vi "BRAM_ReadScoreNumbers.vi"(1 "Number":i16, 4 "Address":i16) -> (16 "PixelData":fxp<+,4,4>)   [LabVIEW 2018]
uses:
  <vilib>/rvi/Memory/Memory_Emulation/nirvimemoryFastEmulation.vi
  <vilib>/rvi/Memory/Memory_Emulation/nirvimemoryEmulation.vi
  <vilib>/rvi/Emulation/niFpgaEmulationIsFPGAContextNoSignature.vi
  <vilib>/rvi/DataTransferAndStorage/Container/Common/niFpgaContainerGetUniqueNameForEmu.vi
  <vilib>/rvi/Emulation/niFpgaProcessEmulError.vi
  <vilib>/rvi/Emulation/niFpgaSctlEmulationGetInTimedLoop.vi
  <vilib>/rvi/errors/nirviReportUnexpectedCaseInternalError (U32).vi
  <vilib>/rvi/DataTransferAndStorage/Container/XNode/niFpgaContainer.xnode
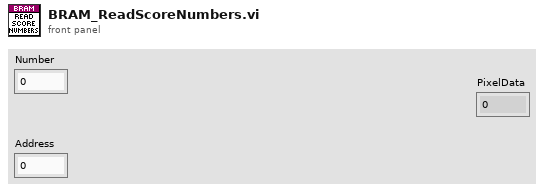
[diagram p1: front panel]
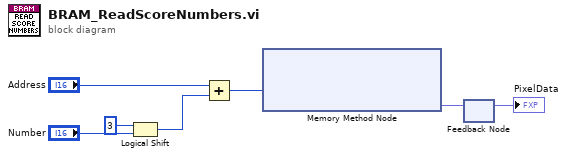
[diagram p0: block diagram]
diagram:
  n1 = Logical Shift(y=i16 3, x="Number") -> (x << y=w1:i16)
  n2 = Add(x="Address", y=w1) -> (x+y=w4:i16)
  n3 = xnode ("Memory Method Node")("Address A"=w4) -> ("Data A"=w7:fxp<+,4,4>)  [unwired: 1 in, 1 out]
  n4 = feedback #1() -> (→"PixelData":fxp<+,4,4>)  [unwired: 1 in]
  n5 = feedback-in #1(w7) -> ()
